vi "PM9_TCP_REMOTE-SET-SETPOINT.vi"(0 "VISA":refnum<visa-resource-name>="TCPIP0::169.254.70.190::502::SOCKET", 5 "connection ID":refnum<k5>, 11 "error in (no error)":errorcluster, 12 "Temp":sgl=25.0 format="%.1g", 14 "Close TCP(t)":bool) -> (4 "visa out":refnum<visa-resource-name>, 6 "connection ID out":refnum<k5>, 15 "error out":errorcluster)   [LabVIEW 2018]
panel:
  # "If in a loop:\nconnect a valid reference\nClose TCP if desired"
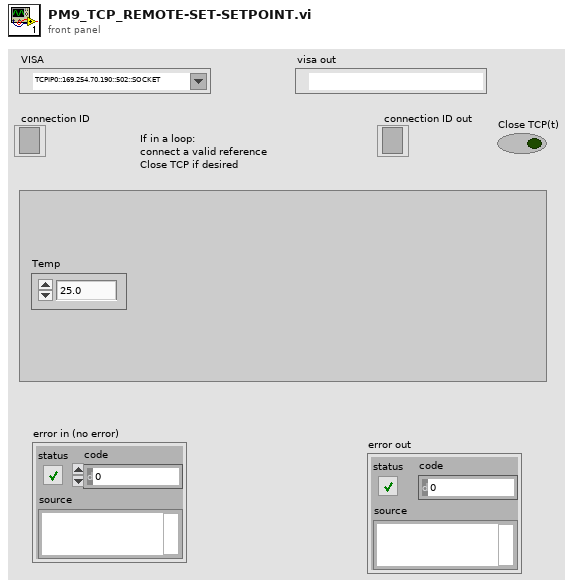
[diagram p1: front panel]
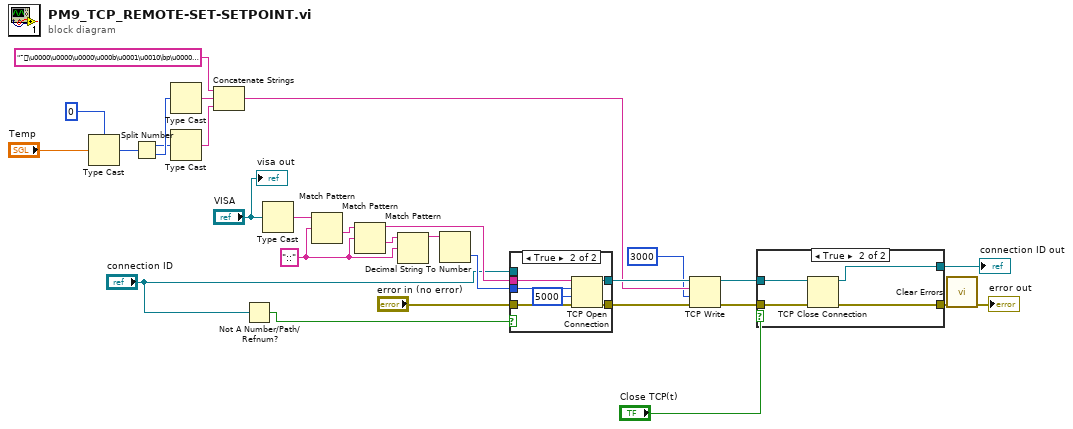
[diagram p0: block diagram]
diagram:
  w11 = "::" ("search string/char (-)")
  n1 = Type Cast(type=0, x="Temp") -> (*(type *) &x=w22:i32)
  n2 = Split Number(x=w22) -> (hi(x)=w20:u16, lo(x)=w21:u16)
  n3 = Type Cast(x=w21) -> (*(type *) &x=w18:string)  [unwired: 1 in]
  n4 = Type Cast(x=w20) -> (*(type *) &x=w17:string)  [unwired: 1 in]
  n5 = Concatenate Strings("¯\u0000\u0000\u0000\u000b\u0001\u0010\bp\u0000\u0002\u0004", w18, w17) -> (w24:string)
  n6 = Not A Number/Path/Refnum?(number/path/refnum="connection ID") -> (NaN/Path/Refnum?=w3:bool)
  n7 = Type Cast(x="VISA") -> (*(type *) &x=w15:string)  [unwired: 1 in]
  n8 = Match Pattern(string=w15, regular expression=w11) -> (after substring=w14:string)  [unwired: 1 in, 3 out]
  n9 = Match Pattern(string=w14, regular expression=w11) -> (before substring=w13:string, after substring=w12:string)  [unwired: 1 in, 2 out]
  n10 = Match Pattern(string=w12, regular expression=w11) -> (before substring=w10:string)  [unwired: 1 in, 3 out]
  n11 = Decimal String To Number(string=w10) -> (number=w9:i32)  [unwired: 2 in, 1 out]
  n12 = case shown="True" w3 {
    tunnel: [w30 w37] -> w29
    tunnel: [w31 w36] -> w28
    tunnel: w13 -> [_ w35]
    tunnel: w9 -> [_ w34]
    tunnel: "error in (no error)" -> [w31 w33]
    tunnel: "connection ID" -> [w30 _]
    frame False {
    }
    frame True {
      n13 = TCP Open Connection(address=w35, remote port or service name=w34, timeout ms (60000)=5000, error in (no error)=w33) -> (connection ID=w37:refnum<k5>, error out=w36:errorcluster)  [unwired: 1 in]
    }
  }
  n14 = TCP Write(connection ID=w29, data in=w24, error in (no error)=w28, 9:3000 ("timeout ms (25000)")) -> (connection ID out=w6:refnum<k5>, error out=w7:errorcluster)  [unwired: 1 out]
  n15 = case shown="True" "Close TCP(t)" {
    tunnel: [w39 w43] -> w27
    tunnel: w7 -> [w39 w42]
    tunnel: w6 -> [w38 w41]
    tunnel: [w38 w40] -> w2
    frame False {
    }
    frame True {
      n16 = TCP Close Connection(connection ID=w41, error in (no error)=w42) -> (connection ID out=w40:refnum<k5>, error out=w43:errorcluster)  [unwired: 1 in]
    }
  }
  "connection ID out" <- w2
  n17 = call <vilib>:"Clear Errors.vi"("error in (no error)"=w27) -> ("error out"=→"error out":errorcluster)  [unwired: 5 in, 1 out]
  "visa out" <- "VISA"
